vi "velosterstack.vi"(11 "VELO_PT_T":T1={"hash"=3444748642197318535, "sys time"=0, "Timestamp"=0, "Rotational angle"=[11547, 11564, 11580, 11596, 11614, 11630, 11647, 11663, 11678, 11696, 11714, 11730], "dist"=[[0, 0, 0, 0, 0, 0, 0, 0, 0, 0, 0, 0, 0, 0, 0, 0, 0, 0, 2933, 2909, 2901, 2913, 2913, 3042, 2913, 2924, 2867, 0, 0, 3082, 0, 4173], [0, 0, 0, 0, 0, 0, 0, 0, 0, 0, 0, 0, 0, 0, 0, 0, 0, 0, 2928, 2906, 2896, 2920, 2914, 3037, 2923, 2919, 2866, 3067, 4160, 4168, 4176, 4183], [0, 0, 0, 0, 0, 0, 0, 0, 0, 0, 0, 0, 0, 0, 0, 0, 0, 0, 2932, 2908, 2900, 2924, 2915, 3046, 2948, 2892, 0, 3056, 4173, 3080, 4176, 4182], [0, 0, 0, 0, 0, 0, 0, 0, 0, 0, 0, 0, 0, 0, 0, 0, 0, 0, 2917, 2916, 2898, 2921, 2926, 3049, 2926, 2890, 2869, 3063, 4175, 4177, 4185, 4181], [0, 0, 0, 0, 0, 0, 0, 0, 0, 0, 0, 0, 0, 0, 0, 0, 0, 0, 2932, 2895, 2917, 2923, 2920, 3056, 2902, 2894, 2873, 0, 3064, 4190, 4187, 4187], [0, 0, 0, 0, 0, 0, 0, 0, 0, 0, 0, 0, 0, 0, 0, 0, 0, 0, 2928, 2908, 2934, 2922, 2922, 3058, 2907, 2902, 2876, 0, 3071, 3087, 4190, 4195], [0, 0, 0, 0, 0, 0, 0, 0, 0, 0, 0, 0, 0, 0, 0, 0, 0, 0, 2921, 2910, 2917, 2920, 2915, 3061, 2903, 2909, 2882, 2984, 3076, 4179, 4197, 4197], [0, 0, 0, 0, 0, 0, 0, 0, 0, 0, 0, 0, 0, 0, 0, 0, 0, 0, 2956, 2909, 3073, 2933, 2944, 3064, 2923, 2914, 2884, 2986, 3083, 4186, 4202, 4204], [0, 0, 0, 0, 0, 0, 0, 0, 0, 0, 0, 0, 0, 0, 0, 0, 0, 0, 2933, 2919, 3070, 2902, 0, 3071, 2917, 2927, 2886, 2991, 3050, 4194, 4205, 4201], [0, 0, 0, 0, 0, 0, 0, 0, 0, 0, 0, 0, 0, 0, 0, 0, 0, 0, 2947, 2918, 3081, 0, 0, 3069, 2930, 2935, 2891, 2994, 0, 4196, 4211, 4216], [0, 0, 0, 0, 0, 0, 0, 0, 0, 0, 0, 0, 0, 0, 0, 0, 0, 0, 2943, 0, 3084, 0, 3048, 3072, 2942, 2929, 2892, 2999, 3049, 4193, 4213, 3113], [0, 0, 0, 0, 0, 0, 0, 0, 0, 0, 0, 0, 0, 0, 0, 0, 0, 0, 2938, 0, 3085, 3045, 3031, 3077, 2942, 2917, 2896, 2999, 3057, 4194, 4217, 3113]], "Intensity"=[[3, 1, 2, 5, 3, 4, 3, 1, 19, 11, 17, 13, 26, 10, 2, 1, 2, 2, 1, 2, 3, 0, 6, 3, 44, 40, 14, 1, 12, 1, 19, 2], [3, 1, 2, 5, 3, 4, 3, 1, 17, 11, 18, 13, 26, 12, 2, 1, 2, 2, 1, 3, 2, 0, 7, 3, 40, 19, 6, 0, 1, 1, 8, 3], [3, 1, 2, 5, 3, 4, 3, 1, 16, 11, 18, 15, 22, 10, 2, 1, 2, 2, 1, 3, 2, 0, 5, 3, 30, 18, 36, 0, 0, 0, 8, 2], [3, 1, 2, 5, 3, 4, 3, 1, 16, 11, 19, 13, 22, 12, 2, 1, 2, 2, 4, 1, 2, 0, 5, 3, 12, 31, 21, 0, 0, 1, 8, 2], [3, 1, 2, 5, 4, 4, 3, 1, 14, 10, 16, 12, 22, 12, 2, 1, 2, 2, 1, 2, 0, 0, 3, 3, 23, 35, 25, 33, 0, 0, 8, 2], [3, 1, 2, 3, 4, 4, 3, 1, 13, 8, 15, 11, 22, 10, 2, 1, 2, 2, 1, 2, 0, 1, 5, 3, 34, 9, 25, 49, 0, 0, 6, 2], [3, 1, 2, 3, 4, 4, 3, 1, 13, 8, 14, 9, 18, 12, 2, 1, 2, 2, 1, 1, 1, 0, 4, 3, 30, 21, 25, 30, 0, 1, 7, 2], [3, 1, 2, 5, 3, 4, 3, 1, 13, 7, 9, 8, 18, 10, 2, 1, 2, 2, 1, 1, 1, 0, 2, 3, 13, 25, 27, 33, 0, 2, 7, 2], [3, 1, 2, 3, 3, 4, 3, 1, 9, 5, 8, 6, 15, 8, 2, 1, 2, 2, 1, 2, 1, 0, 28, 3, 26, 14, 25, 39, 2, 2, 7, 2], [3, 1, 2, 3, 3, 3, 3, 1, 6, 5, 7, 5, 15, 8, 2, 1, 2, 2, 1, 0, 1, 1, 64, 3, 38, 15, 27, 44, 42, 2, 7, 1], [3, 1, 2, 3, 3, 3, 3, 1, 6, 5, 4, 5, 15, 8, 2, 1, 2, 2, 1, 2, 1, 1, 8, 3, 34, 15, 23, 42, 5, 2, 7, 0], [3, 1, 2, 5, 3, 3, 3, 1, 6, 5, 4, 5, 15, 8, 2, 1, 2, 2, 1, 2, 1, 0, 2, 3, 40, 18, 23, 42, 3, 2, 7, 0]], "pos_x"=0.0, "pos_y"=0.0, "pos_h"=0.0}) -> (3 "updated":bool)   [LabVIEW 2015]
uses:
  G_SEN.vi
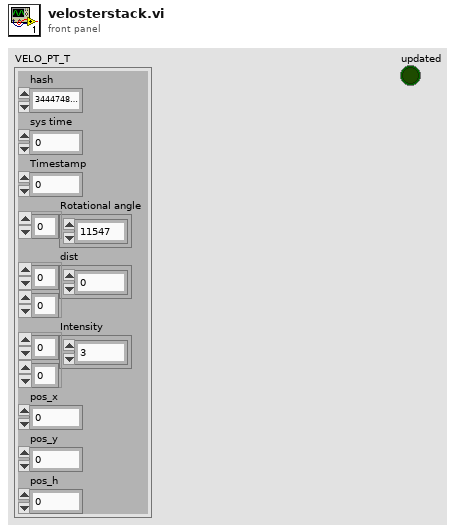
[diagram p1: front panel]
types:
  T1 = cluster{"hash":i64, "sys time":i64, "Timestamp":u32, "Rotational angle":u16[], "dist":u16[][], "Intensity":u8[][], "pos_x":dbl, "pos_y":dbl, "pos_h":dbl}
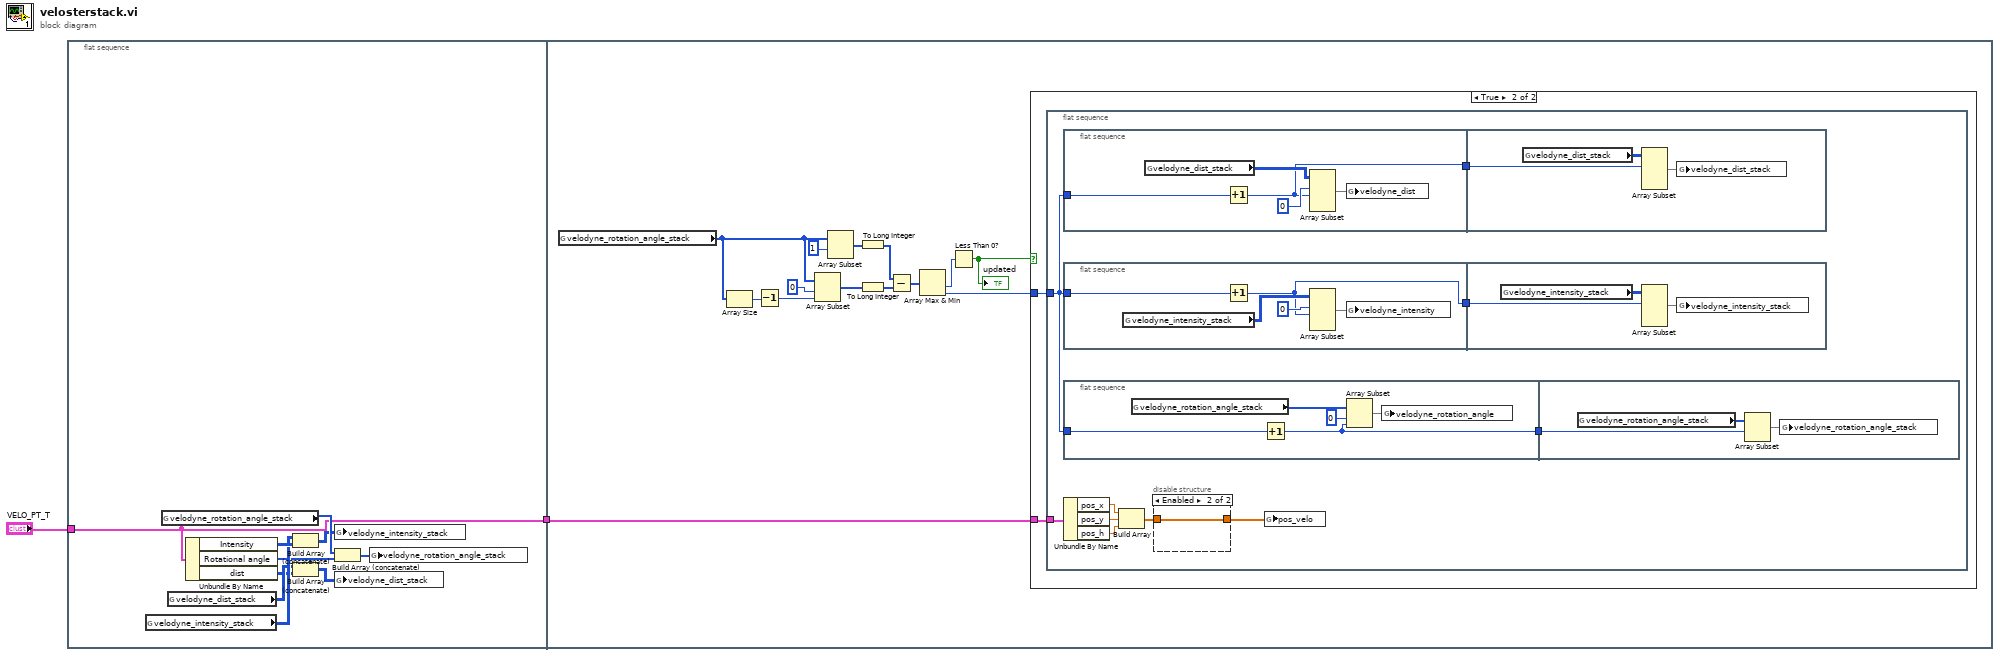
[diagram p0: block diagram]
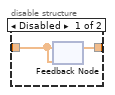
[diagram p3: hidden frame]
diagram:
  n1 = flat-sequence {
    tunnel: "VELO_PT_T" -> [w3]
    tunnel: [w3] -> w1
    tunnel: w1 -> [w13]
    frame #0 {
      n2 = global read "G_SEN.vi" "velodyne_intensity_stack"() -> (w8:u8[][])
      n3 = global read "G_SEN.vi" "velodyne_rotation_angle_stack"() -> (w12:u16[])
      n4 = global read "G_SEN.vi" "velodyne_dist_stack"() -> (w7:u16[][])
      n5 = Unbundle By Name(w3) -> ("Intensity"=w9:u8[][], "Rotational angle"=w5:u16[], "dist"=w4:u16[][])
      n6 = Build Array (concatenate)(w8, w9) -> (w10:u8[][])
      n7 = Build Array (concatenate)(w7, w4) -> (w6:u16[][])
      n8 = global write "G_SEN.vi" "velodyne_intensity_stack"(w10) -> ()
      n9 = Build Array (concatenate)(w12, w5) -> (w11:u16[])
      n10 = global write "G_SEN.vi" "velodyne_dist_stack"(w6) -> ()
      n11 = global write "G_SEN.vi" "velodyne_rotation_angle_stack"(w11) -> ()
    }
    frame #1 {
      n12 = global read "G_SEN.vi" "velodyne_rotation_angle_stack"() -> (w15:u16[])
      n13 = Array Size(array=w15) -> (size(s)=w26:i32)
      n14 = Decrement(x=w26) -> (x-1=w25:i32)
      n15 = Array Subset(array=w15, index=0, length=w25) -> (w21:u16[])
      n16 = Array Subset(array=w15, index=1) -> (w22:u16[])  [unwired: 1 in]
      n17 = To Long Integer(number=w22) -> (32bit integer=w20:i32[])
      n18 = To Long Integer(number=w21) -> (32bit integer=w19:i32[])
      n19 = Subtract(x=w20, y=w19) -> (x-y=w18:i32[])
      n20 = Array Max & Min(array=w18) -> (min value=w17:i32, min index (indices)=w16:i32)  [unwired: 2 out]
      n21 = Less Than 0?(x=w17) -> (x < 0?=w14:bool)
      "updated" <- w14
      n22 = case shown="True" w14 {
        tunnel: w16 -> [_ w28]
        tunnel: w13 -> [_ w27]
        frame False {
        }
        frame True {
          n23 = flat-sequence {
            tunnel: w28 -> [w35]
            tunnel: w27 -> [w34]
            frame #0 {
              n24 = flat-sequence {
                tunnel: w35 -> [w52]
                tunnel: [w50] -> w37
                tunnel: w37 -> [w55]
                frame #0 {
                  n25 = global read "G_SEN.vi" "velodyne_dist_stack"() -> (w54:u16[][])
                  n26 = Increment(x=w52) -> (x+1=w50:i32)
                  n27 = Array Subset(array=w54, index (row)=0 ("index"), length (row)=w50) -> (w51:u16[][])  [unwired: 2 in]
                  n28 = global write "G_SEN.vi" "velodyne_dist"(w51) -> ()
                }
                frame #1 {
                  n29 = global read "G_SEN.vi" "velodyne_dist_stack"() -> (w57:u16[][])
                  n30 = Array Subset(array=w57, index (row)=w55) -> (w56:u16[][])  [unwired: 3 in]
                  n31 = global write "G_SEN.vi" "velodyne_dist_stack"(w56) -> ()
                }
              }
              n32 = flat-sequence {
                tunnel: w35 -> [w44]
                tunnel: [w42] -> w36
                tunnel: w36 -> [w47]
                frame #0 {
                  n33 = global read "G_SEN.vi" "velodyne_intensity_stack"() -> (w46:u8[][])
                  n34 = Increment(x=w44) -> (x+1=w42:i32)
                  n35 = Array Subset(array=w46, index (row)=0 ("index"), length (row)=w42) -> (w43:u8[][])  [unwired: 2 in]
                  n36 = global write "G_SEN.vi" "velodyne_intensity"(w43) -> ()
                }
                frame #1 {
                  n37 = global read "G_SEN.vi" "velodyne_intensity_stack"() -> (w49:u8[][])
                  n38 = Array Subset(array=w49, index (row)=w47) -> (w48:u8[][])  [unwired: 3 in]
                  n39 = global write "G_SEN.vi" "velodyne_intensity_stack"(w48) -> ()
                }
              }
              n40 = flat-sequence {
                tunnel: w35 -> [w60]
                tunnel: [w58] -> w38
                tunnel: w38 -> [w63]
                frame #0 {
                  n41 = global read "G_SEN.vi" "velodyne_rotation_angle_stack"() -> (w62:u16[])
                  n42 = Increment(x=w60) -> (x+1=w58:i32)
                  n43 = Array Subset(array=w62, index=0, length=w58) -> (w59:u16[])
                  n44 = global write "G_SEN.vi" "velodyne_rotation_angle"(w59) -> ()
                }
                frame #1 {
                  n45 = global read "G_SEN.vi" "velodyne_rotation_angle_stack"() -> (w65:u16[])
                  n46 = Array Subset(array=w65, index=w63) -> (w64:u16[])  [unwired: 1 in]
                  n47 = global write "G_SEN.vi" "velodyne_rotation_angle_stack"(w64) -> ()
                }
              }
              n48 = Unbundle By Name(w34) -> ("pos_x"=w33:dbl, "pos_y"=w32:dbl, "pos_h"=w31:dbl)
              n49 = Build Array(w33, w32, w31) -> (w30:dbl[])
              n50 = disable-structure shown="Enabled" {
                disable-tunnel: w30 -> [w40 w41]
                disable-tunnel: [w39 w41] -> w29
                frame Disabled {
                  n51 = feedback #1(w40) -> (w39:dbl[])
                  n52 = feedback-in #1(w40) -> ()
                }
                frame Enabled {
                }
              }
              n53 = global write "G_SEN.vi" "pos_velo"(w29) -> ()
            }
          }
        }
      }
    }
  }
